vi "Station2_Data_Log.vi"(8 "error in (no error)":errorcluster, 11 "Cluster":T2) -> (0 "error out":errorcluster)   [LabVIEW 2017]
uses:
  <vilib>/addons/database/Connection.llb/Conn ObjectReference.ctl
  <vilib>/addons/database/NI_Database_API.lvlib
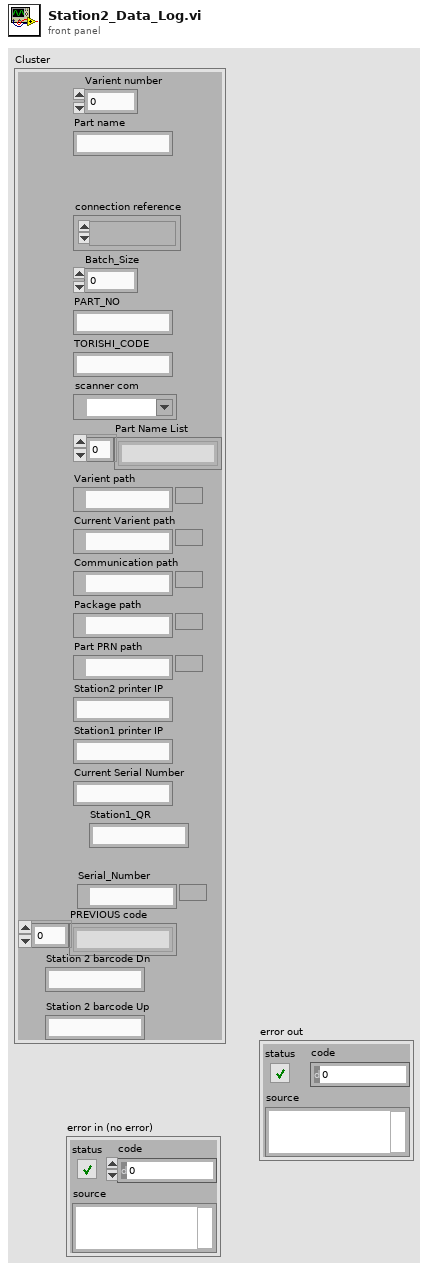
[diagram p1: front panel]
types:
  T1 = typedef "NI_Database_API.lvlib/Conn ObjectReference.ctl" = refnum<k1>
  T2 = cluster{"Varient number":u16, "Part name":string, "connection reference":T1, "Batch_Size":u16, "PART_NO":string, "TORISHI_CODE":string, "scanner com":refnum<visa-resource-name>, "Part Name List":string[], "Varient path":path, "Current Varient path":path, "Communication path":path, "Package path":path, "Part PRN path":path, "Station2 printer IP":string, "Station1 printer IP":string, "Current Serial Number":string, "Station1_QR":string, "Serial_Number":path, "PREVIOUS code":string[], "Station 2 barcode Dn":string, "Station 2 barcode Up":string}
  T3 = cluster{string, "Station 2 barcode Up":string, "Station 2 barcode Dn":string}
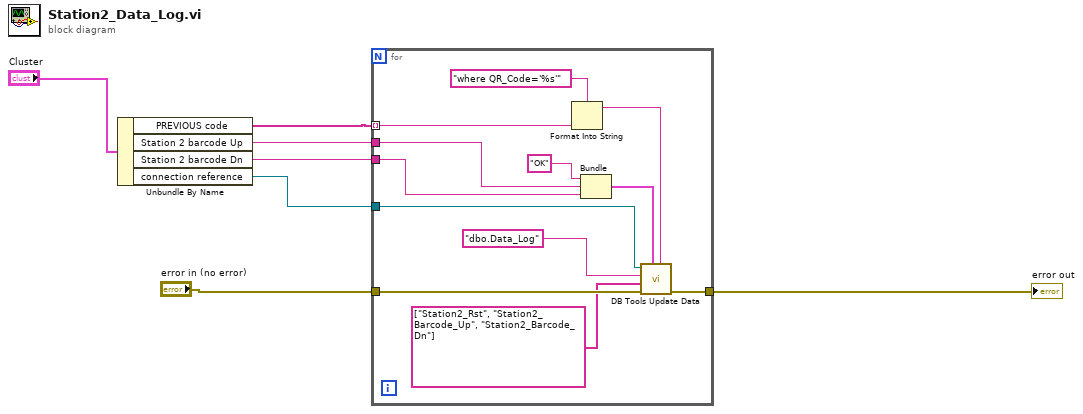
[diagram p0: block diagram]
diagram:
  n1 = Unbundle By Name("Cluster") -> ("PREVIOUS code"=w4:string[], "Station 2 barcode Up"=w3:string, "Station 2 barcode Dn"=w2:string, "connection reference"=w1:T1)
  n2 = for {
    tunnel: [w18] -> w6
    tunnel: w1 -> [w17]
    tunnel: "error in (no error)" -> [w14]
    tunnel: w4 -> [w12] mode=indexing
    tunnel: w3 -> [w10]
    tunnel: w2 -> [w9]
    n3 = Format Into String(format string="where QR_Code='%s'", w12) -> (resulting string=w11:string)  [unwired: 2 in, 1 out]
    n4 = Bundle("OK", "Station 2 barcode Up"=w10, "Station 2 barcode Dn"=w9) -> (w15:T3)  [unwired: 1 in]
    n5 = call <vilib>:"DB Tools Update Data.vi"("condition"=w11, "data"=w15, "error in (no error)"=w14, "columns"=string[] ["Station2_Rst", "Station2_Barcode_Up", "Station2_Barcode_Dn"] ("columns 2"), "table"="dbo.Data_Log", "connection reference"=w17) -> ("error out"=w18:errorcluster)  [unwired: 4 in, 1 out]
  }
  "error out" <- w6
